vi "CargoStateControl.vi"(9 "Elevator State":string="Cargo_Feeder") -> ()   [LabVIEW 2018]
uses:
  RobotStates.vi
  Inputs_DriverStation.vi
  SensorReadings.vi
panel:
  in  "Threshold (ms)":u32=300
  in  "Current Threshold (A)":dbl=20.0
  in  "Current Ignore Time (ms)":u32=1000
  out "Intake Velocity":dbl
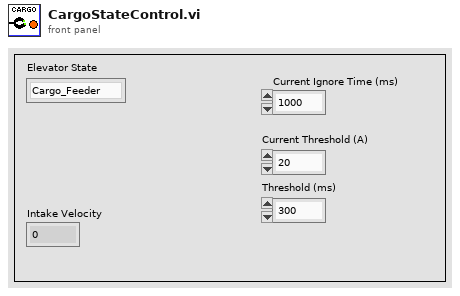
[diagram p1: front panel]
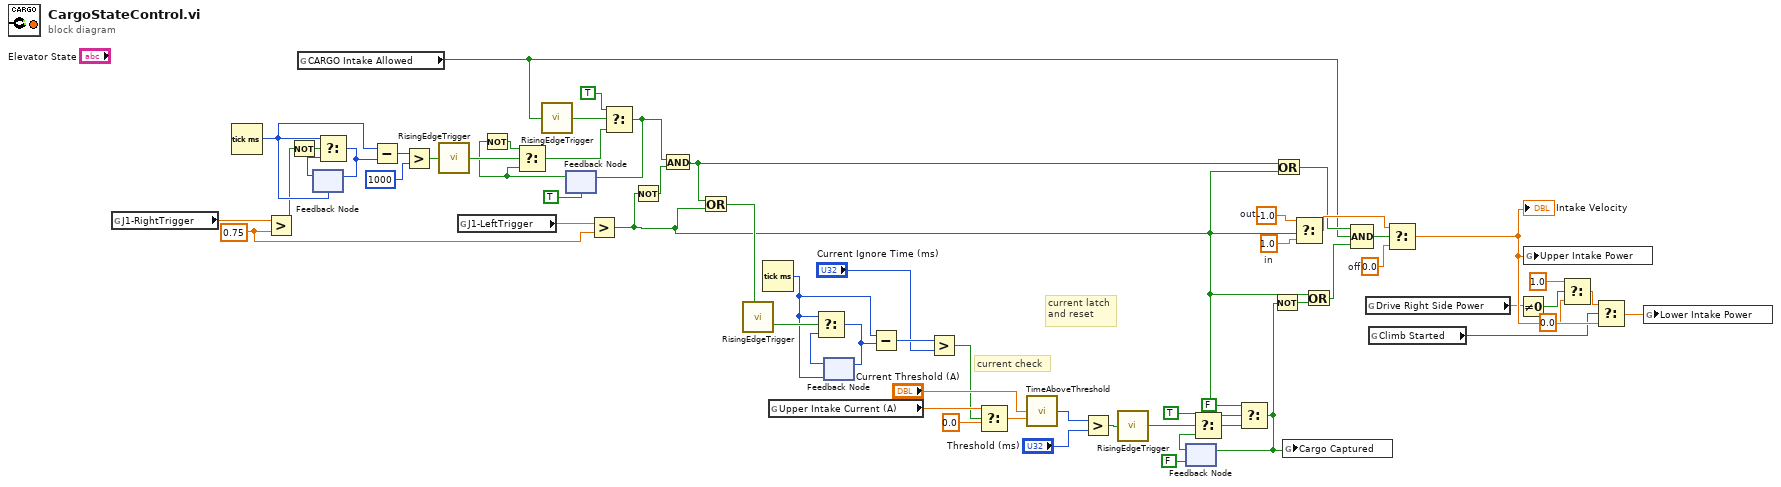
[diagram p0: block diagram]
diagram:
  w50 = 0.75 ("y")
  w58 = 0.0  # off
  w59 = 1.0  # in
  w60 = -1.0  # out
  # "current check"
  # "current latch\nand reset"
  n1 = global read "Inputs_DriverStation.vi" "J1-RightTrigger"() -> (w49:dbl)
  n2 = Tick Count (ms)() -> (millisecond timer value=w5:u32)
  n3 = Greater?(x=w49, y=w50) -> (0:w3:bool)
  n4 = Not(x=w3) -> (.not. x?=w1:bool)
  n5 = global read "RobotStates.vi" "CARGO Intake Allowed"() -> (w25:bool)
  n6 = feedback #1(w5) -> (w4:u32)
  n7 = Select(t=w5, s=w1, f=w4) -> (s? t:f=w6:u32)
  n8 = feedback-in #1(w6) -> ()
  n9 = Subtract(x=w5, y=w6) -> (x-y=w7:u32)
  n10 = Greater?(x=w7, y=u32 1000) -> (0:w2:bool)
  n11 = call "RisingEdgeTrigger.vi"("Raw Signal"=w2) -> ("Trigger"=w19:bool)
  n12 = global read "Inputs_DriverStation.vi" "J1-LeftTrigger"() -> (w48:dbl)
  n13 = call "RisingEdgeTrigger.vi"("Raw Signal"=w25) -> ("Trigger"=w24:bool)
  n14 = feedback #2(TRUE) -> (w17:bool)
  n15 = Not(x=w17) -> (.not. x?=w18:bool)
  n16 = Select(t=w18, s=w19, f=w17) -> (s? t:f=w20:bool)
  n17 = Greater?(x=w48, y=w50) -> (0:w28:bool)
  n18 = Select(t=TRUE, s=w24, f=w20) -> (s? t:f=w22:bool)
  n19 = feedback-in #2(w22) -> ()
  n20 = Not(x=w28) -> (.not. x?=w27:bool)
  n21 = And(x=w22, y=w27) -> (x .and. y?=w26:bool)
  n22 = Or(x=w26, y=w28) -> (x .or. y?=w46:bool)
  n23 = call "RisingEdgeTrigger.vi"("Raw Signal"=w46) -> ("Trigger"=w45:bool)
  n24 = Tick Count (ms)() -> (millisecond timer value=w42:u32)
  n25 = global read "SensorReadings.vi" "Upper Intake Current (A)"() -> (w33:dbl)
  n26 = feedback #3(w42) -> (w44:u32)
  n27 = Select(t=w42, s=w45, f=w44) -> (s? t:f=w43:u32)
  n28 = feedback-in #3(w43) -> ()
  n29 = Subtract(x=w42, y=w43) -> (x-y=w41:u32)
  n30 = Greater?(x=w41, y="Current Ignore Time (ms)") -> (0:w30:bool)
  n31 = Select(t=w33, s=w30, f=0.0) -> (s? t:f=w31:dbl)
  n32 = call "TimeAboveThreshold.vi"("Current Value"=w31, "Threshold"="Current Threshold (A)") -> ("Time Above"=w37:u32)  [unwired: 3 in]
  n33 = Greater?(x=w37, y="Threshold (ms)") -> (0:w35:bool)
  n34 = call "RisingEdgeTrigger.vi"("Raw Signal"=w35) -> ("Trigger"=w36:bool)
  n35 = feedback #4(FALSE ("t")) -> (w55:bool)
  n36 = Select(t=TRUE, s=w36, f=w55) -> (s? t:f=w54:bool)
  n37 = Select(t=FALSE, s=w28, f=w54) -> (s? t:f=w47:bool)
  n38 = feedback-in #4(w47) -> ()
  n39 = Not(x=w47) -> (.not. x?=w57:bool)
  n40 = Or(x=w26, y=w28) -> (x .or. y?=w39:bool)
  n41 = global write "SensorReadings.vi" "Cargo Captured"(w47) -> ()
  n42 = Select(t=w60, s=w28, f=w59) -> (s? t:f=w61:dbl)
  n43 = Or(x=w28, y=w57) -> (x .or. y?=w51:bool)
  n44 = Compound Arithmetic op=AND(w39, w25, w51) -> (w52:bool)
  n45 = global read "RobotStates.vi" "Drive Right Side Power"() -> (w13:dbl)
  n46 = global read "RobotStates.vi" "Climb Started"() -> (w15:bool)
  n47 = Select(t=w61, s=w52, f=w58) -> (s? t:f=w16:dbl)
  "Intake Velocity" <- w16
  n48 = Not Equal To 0?(x=w13) -> (x != 0?=w12:bool)
  n49 = global write "RobotStates.vi" "Upper Intake Power"(w16) -> ()
  n50 = Select(t=1.0, s=w12, f=0.0) -> (s? t:f=w9:dbl)
  n51 = Select(t=w9, s=w15, f=w16) -> (s? t:f=w14:dbl)
  n52 = global write "RobotStates.vi" "Lower Intake Power"(w14) -> ()
